vi "Open.vi"(7 "Allow multiple opens?":bool, 8 "error in (no error)":errorcluster, 10 "Channel Names":tag[](array[tag])) -> (0 "error out":errorcluster, 3 "Accelerometer Ref Out":T1)   [LabVIEW 2021, in "Accelerometer.lvlib"]
doc: "Opens a reference to one or more accelerometer channels. You must open a reference before you read values from an accelerometer channel."
uses:
  <vilib>/myRIO/Instrument Drivers/Onboard Devices/Accelerometer/Accelerometer.lvlib
  <vilib>/myRIO/Instrument Drivers/Onboard Devices/Accelerometer/typedefs/Accelerometer Reference.ctl
  <vilib>/myRIO/Common/Instrument Driver Framework/Utilities/typedefs/myRIO Generic Hardware Reference.ctl
  <vilib>/myRIO/Common/Instrument Driver Framework/Utilities/typedefs/Hardware Version Enum.ctl
  <vilib>/myRIO/Common/Instrument Driver Framework/Utilities/typedefs/myRIO v1.0 Reference.ctl
  <vilib>/myRIO/Common/Instrument Driver Framework/Utilities/typedefs/Generic FPGA Reference.ctl
  <vilib>/myRIO/Common/Instrument Driver Framework/myRIO v1.0/Accelerometer/typedefs/Accelerometer Channels List.ctl
  <vilib>/myRIO/Common/Instrument Driver Framework/myRIO v1.0/Accelerometer/typedefs/Accelerometer Channels Enum.ctl
  <vilib>/myRIO/Common/Instrument Driver Framework/Utilities/vis/Validate Channels.vi
  <vilib>/myRIO/Common/Instrument Driver Framework/myRIO v1.0/Accelerometer/vis/myRIO v1.0 Reserve Accelerometer.vi
  <vilib>/myRIO/Common/Instrument Driver Framework/roboRIO v1.0/Accelerometer/vis/roboRIO v1.0 Reserve Accelerometer.vi
  <vilib>/myRIO/Common/Instrument Driver Framework/myRIO v1.0/Resource Manager/vis/myRIO v1.0 Reserve Channel List.vi
  <vilib>/myRIO/Common/Instrument Driver Framework/myRIO v1.0/Accelerometer/vis/myRIO v1.0 Build MUX Configuration Accelerometer.vi
  <vilib>/myRIO/Common/Instrument Driver Framework/roboRIO v1.0/Resource Manager/vis/roboRIO v1.0 Reserve Channel List.vi
  <vilib>/myRIO/Common/Instrument Driver Framework/roboRIO v1.0/Accelerometer/vis/roboRIO v1.0 Build MUX Configuration Accelerometer.vi
  <vilib>/myRIO/Common/Instrument Driver Framework/myRIO v1.0/Resource Manager/vis/myRIO v1.0 Reserve Channel.vi
  <vilib>/myRIO/Common/Instrument Driver Framework/myRIO v1.0/Resource Manager/vis/myRIO v1.0 Unreserve Channel.vi
  <vilib>/myRIO/Common/Instrument Driver Framework/roboRIO v1.0/Resource Manager/vis/roboRIO v1.0 Reserve Channel.vi
  <vilib>/myRIO/Common/Instrument Driver Framework/roboRIO v1.0/Resource Manager/vis/roboRIO v1.0 Unreserve Channel.vi
  <vilib>/myRIO/Common/Instrument Driver Framework/myRIO v1.0/Resource Manager/vis/myRIO v1.0 Build Mutex Name.vi
  <vilib>/myRIO/Common/Instrument Driver Framework/roboRIO v1.0/Resource Manager/vis/roboRIO v1.0 Build Mutex Name.vi
  <vilib>/Utility/VariantDataType/GetNumericInfo.vi
  <vilib>/myRIO/Common/Instrument Driver Framework/myRIO v1.0/Accelerometer/vis/myRIO v1.0 Get Scaling Constant Accelerometer.vi
  <vilib>/myRIO/Common/Instrument Driver Framework/Utilities/vis/IO Manager.vi
  <vilib>/myRIO/Common/Instrument Driver Framework/Utilities/vis/Configuration Manager.vi
  <vilib>/myRIO/Common/Instrument Driver Framework/myRIO v1.0/myRIO v1.0 Close.vi
  <vilib>/myRIO/Common/Instrument Driver Framework/roboRIO v1.0/Accelerometer/vis/roboRIO v1.0 Get Scaling Constant Accelerometer.vi
  <vilib>/userdefined/High Color/nirio_resource_hc.ctl
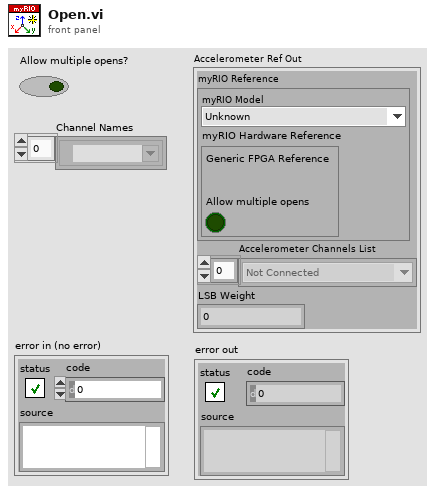
[diagram p1: front panel]
types:
  T1 = typedef "Accelerometer.lvlib/Accelerometer Reference.ctl" = cluster{"myRIO Reference":T2, "Accelerometer Channels List":T6, "LSB Weight":dbl}
  T2 = typedef "myRIO Generic Hardware Reference.ctl" = cluster{"myRIO Model":T3, "myRIO Hardware Reference":T4}
  T3 = typedef "Hardware Version Enum.ctl" = enum16{"Unknown", "myRIO-1900", "myRIO-1950", "roboRIO", "NI ELVIS RIO CM", "ELVIS III"}
  T4 = typedef "myRIO v1.0 Reference.ctl" = cluster{"Generic FPGA Reference":T5, "Allow multiple opens":bool}
  T5 = typedef "Generic FPGA Reference.ctl" = refnum<k20>
  T6 = typedef "Accelerometer Channels List.ctl" = T7[]
  T7 = typedef "Accelerometer Channels Enum.ctl" = enum16{"Not Connected", "X-Axis", "Y-Axis", "Z-Axis"}
  T8 = typedef "nirio_resource_hc.ctl" = tag
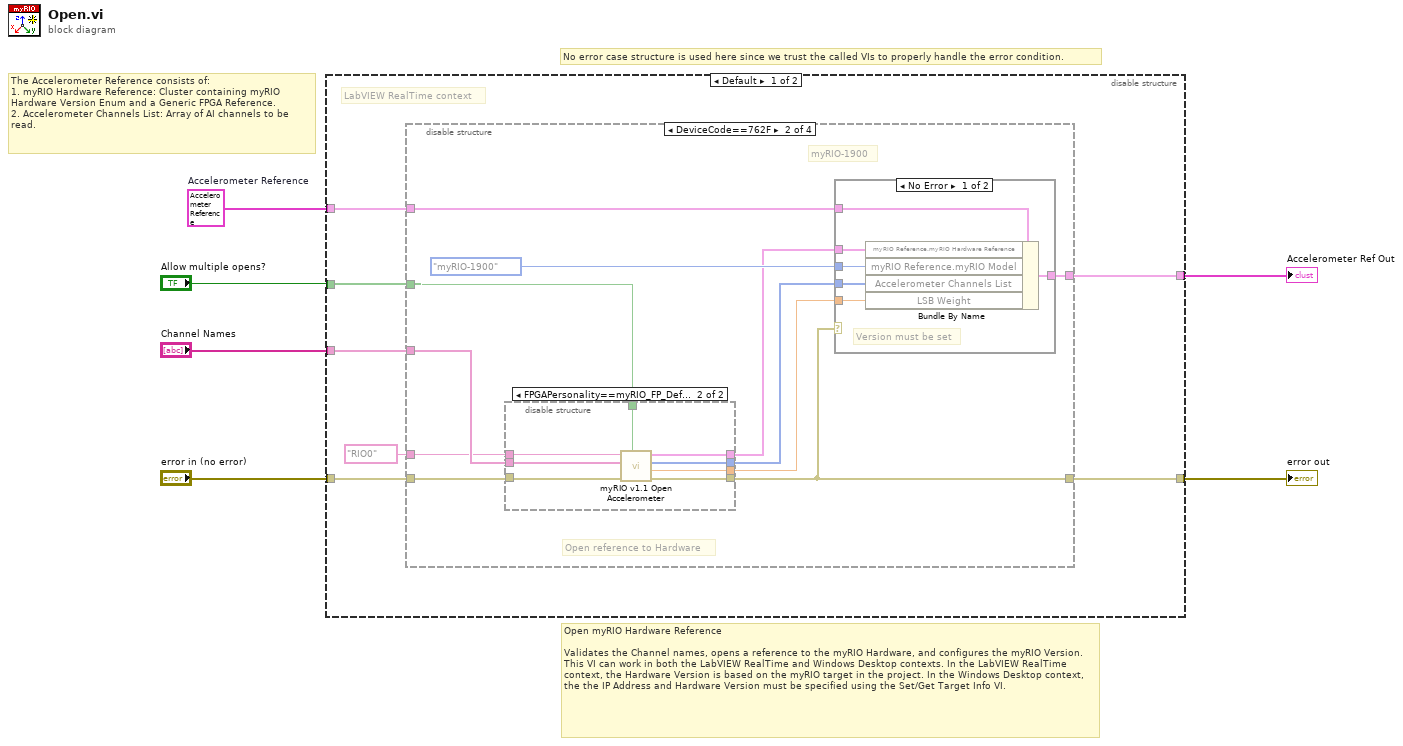
[diagram p0: block diagram]
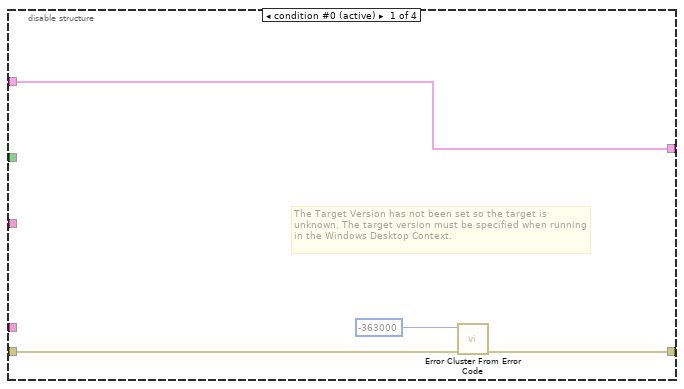
[diagram p2: hidden frame]
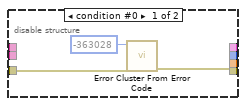
[diagram p3: hidden frame]
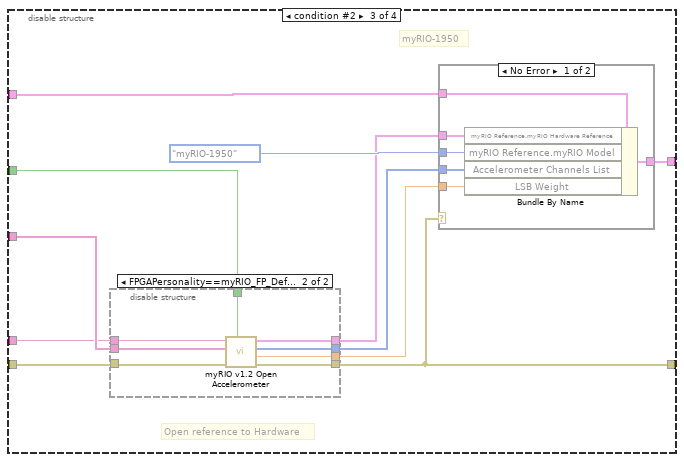
[diagram p5: hidden frame]
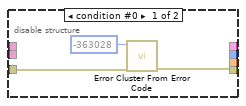
[diagram p6: hidden frame]
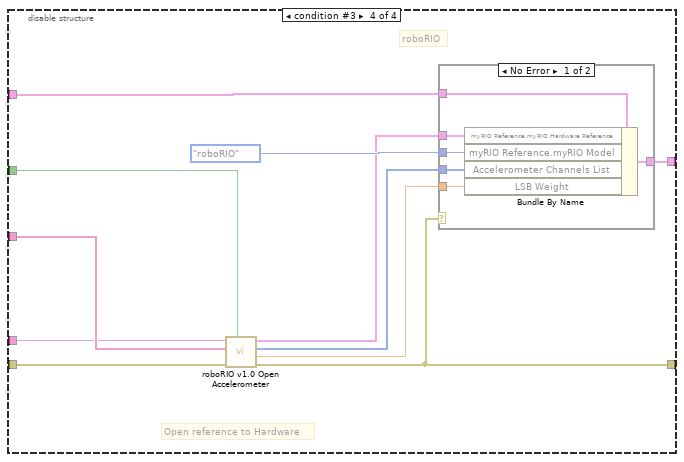
[diagram p8: hidden frame]
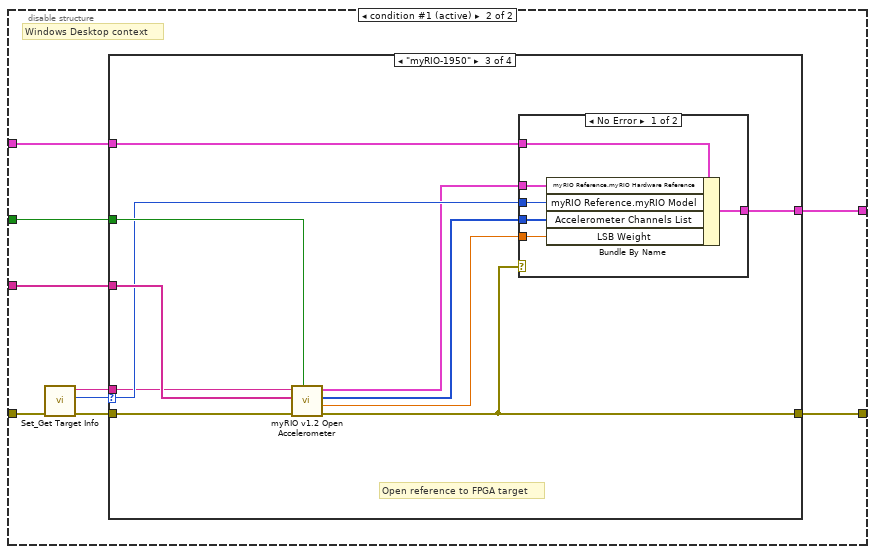
[diagram p10: hidden frame]
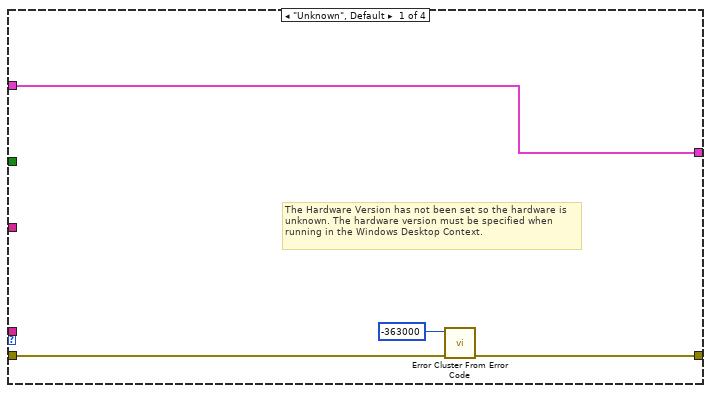
[diagram p11: hidden frame]
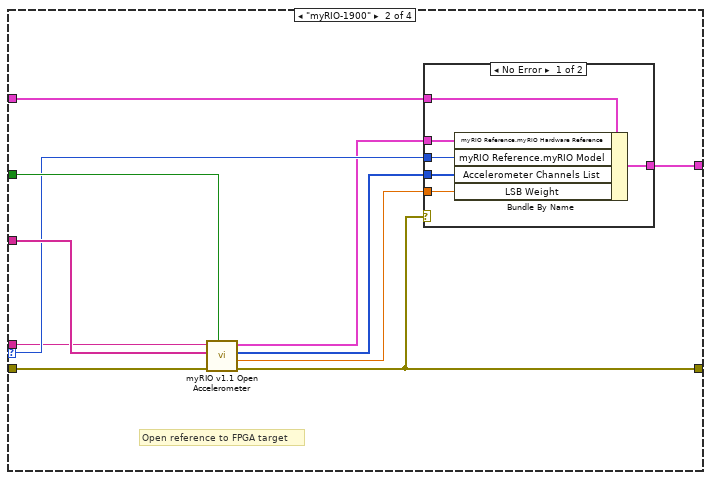
[diagram p12: hidden frame]
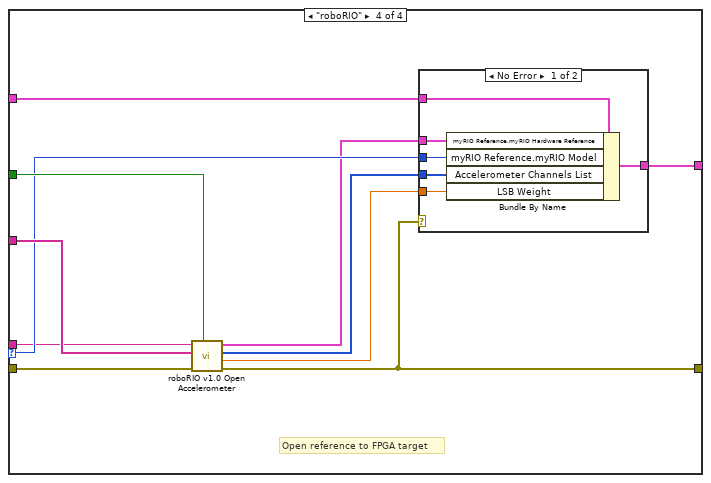
[diagram p15: hidden frame]
diagram:
  w3 = T1 {"myRIO Reference"={"myRIO Model"=enum."Unknown", "myRIO Hardware Reference"={"Generic FPGA Reference"=refnum, "Allow multiple opens"=FALSE}}, "Accelerometer Channels List"=[], "LSB Weight"=0.0}  # Accelerometer Reference
  # "No error case structure is used here since we trust the called VIs to properly handle the error condition."
  # "The Accelerometer Reference consists of:\n1. myRIO Hardware Reference: Cluster containing myRIO Hardware Version Enum and a Generic FPGA Reference.\n2. Accelerometer Channels List: Array of AI channels to be read."
  # "Open myRIO Hardware Reference\n\nValidates the Channel names, opens a reference to the myRIO Hardware, and configures the myRIO Version. This VI can work in both the LabVIEW RealTime and Windows Desktop contexts. In the LabVIEW RealTime context, the Hardware Version is based on the myRIO target in the project. In the Windows Desktop context, the the IP Address and Hardware Version must be specified using the Set/Get Target Info VI."
  n1 = disable-structure shown="Default" {
    disable-tunnel: [w13 w101] -> w4
    disable-tunnel: "Channel Names" -> [w12 w98]
    disable-tunnel: "Allow multiple opens?" -> [w11 w100]
    disable-tunnel: [w10 w99] -> w2
    disable-tunnel: "error in (no error)" -> [w9 w97]
    disable-tunnel: w3 -> [w8 w96]
    frame condition #0 {
      # "LabVIEW RealTime context"
      n2 = disable-structure shown="DeviceCode==762F" {
        disable-tunnel: [w17 w20 w48 w77] -> w13
        disable-tunnel: w12 -> [_ w28 w57 w86]
        disable-tunnel: w11 -> [_ w24 w56 w85]
        disable-tunnel: [w14 w27 w55 w84] -> w10
        disable-tunnel: w9 -> [w16 w25 w53 w82]
        disable-tunnel: w8 -> [w14 w23 w51 w80]
        disable-tunnel: T8 "RIO0" ("Resource name") -> [_ w21 w49 w78]
        frame condition #0 (active) {
          # "The Target Version has not been set so the target is unknown. The target version must be specified when running in the Windows Desktop Context."
          n3 = call <vilib>:"Error Cluster From Error Code.vi"("error in (no error)"=w16, "error code (0)"=-363000) -> ("error out"=w17:errorcluster)  [unwired: 7 in]
        }
        frame condition #1 {
          # "myRIO-1900"
          # "Open reference to Hardware"
          n4 = disable-structure shown="FPGAPersonality==myRIO_FP_Default, Default" {
            disable-tunnel: w28 -> [_ w39]
            disable-tunnel: w25 -> [w30 w38]
            disable-tunnel: w24 -> [_ w37]
            disable-tunnel: [_ w36] -> w22
            disable-tunnel: w21 -> [_ w35]
            disable-tunnel: [w29 w34] -> w20
            disable-tunnel: [_ w33] -> w19
            disable-tunnel: [_ w32] -> w18
            frame condition #0 {
              n5 = call <vilib>:"Error Cluster From Error Code.vi"("error in (no error)"=w30, "error code (0)"=-363028) -> ("error out"=w29:errorcluster)  [unwired: 7 in]
            }
            frame condition #1 (active) {
              n6 = call <vilib>:"myRIO v1.1 Open Accelerometer.vi"("Allow multiple opens?"=w37, "error in (no error)"=w38, "Channel Names"=w39, "Resource name"=w35) -> ("error out"=w34:errorcluster, "LSB Weight"=w32:dbl, "Accelerometer Channel List"=w36:T6, "myRIO Ref Out"=w33:T4)  [unwired: 4 in]
            }
          }
          n7 = case shown="No Error" w20 {
            tunnel: [w45 w46] -> w27
            tunnel: Hardware_Version_Enum."myRIO-1900" ("Hardware Version Enum") -> [w44 _]
            tunnel: w23 -> [w43 w46]
            tunnel: w22 -> [w42 _]
            tunnel: w19 -> [w41 _]
            tunnel: w18 -> [w40 _]
            frame No Error {
              # "Version must be set"
              n8 = Bundle By Name(cluster=w43, "myRIO Reference.myRIO Hardware Reference"=w41, "myRIO Reference.myRIO Model"=w44, "Accelerometer Channels List"=w42, "LSB Weight"=w40) -> (w45:T1)
            }
            frame Error {
            }
          }
        }
        frame condition #2 {
          # "myRIO-1950"
          # "Open reference to Hardware"
          n9 = disable-structure shown="FPGAPersonality==myRIO_FP_Default, Default" {
            disable-tunnel: w57 -> [_ w68]
            disable-tunnel: w56 -> [_ w67]
            disable-tunnel: w53 -> [w59 w66]
            disable-tunnel: [_ w65] -> w52
            disable-tunnel: [_ w64] -> w50
            disable-tunnel: w49 -> [_ w63]
            disable-tunnel: [w58 w62] -> w48
            disable-tunnel: [_ w61] -> w47
            frame condition #0 {
              n10 = call <vilib>:"Error Cluster From Error Code.vi"("error in (no error)"=w59, "error code (0)"=-363028) -> ("error out"=w58:errorcluster)  [unwired: 7 in]
            }
            frame condition #1 (active) {
              n11 = call <vilib>:"myRIO v1.2 Open Accelerometer.vi"("Allow multiple opens?"=w67, "error in (no error)"=w66, "Channel Names"=w68, "Resource name"=w63) -> ("error out"=w62:errorcluster, "LSB Weight"=w61:dbl, "Accelerometer Channel List"=w64:T6, "myRIO Ref Out"=w65:T4)  [unwired: 4 in]
            }
          }
          n12 = case shown="No Error" w48 {
            tunnel: [w74 w75] -> w55
            tunnel: Hardware_Version_Enum."myRIO-1950" ("Hardware Version Enum") -> [w73 _]
            tunnel: w52 -> [w70 _]
            tunnel: w51 -> [w72 w75]
            tunnel: w50 -> [w71 _]
            tunnel: w47 -> [w69 _]
            frame No Error {
              n13 = Bundle By Name(cluster=w72, "myRIO Reference.myRIO Hardware Reference"=w70, "myRIO Reference.myRIO Model"=w73, "Accelerometer Channels List"=w71, "LSB Weight"=w69) -> (w74:T1)
            }
            frame Error {
            }
          }
        }
        frame condition #3 {
          # "roboRIO"
          # "Open reference to Hardware"
          n14 = call <vilib>:"roboRIO v1.0 Open Accelerometer.vi"("Allow multiple opens?"=w85, "error in (no error)"=w82, "Channel Names"=w86, "Resource name"=w78) -> ("error out"=w77:errorcluster, "LSB Weight"=w76:dbl, "Accelerometer Channel List"=w79:T6, "myRIO Ref Out"=w81:T4)  [unwired: 4 in]
          n15 = case shown="No Error" w77 {
            tunnel: [w92 w93] -> w84
            tunnel: Hardware_Version_Enum."roboRIO" ("Hardware Version Enum") -> [w91 _]
            tunnel: w81 -> [w88 _]
            tunnel: w80 -> [w90 w93]
            tunnel: w79 -> [w89 _]
            tunnel: w76 -> [w87 _]
            frame No Error {
              n16 = Bundle By Name(cluster=w90, "myRIO Reference.myRIO Hardware Reference"=w88, "myRIO Reference.myRIO Model"=w91, "Accelerometer Channels List"=w89, "LSB Weight"=w87) -> (w92:T1)
            }
            frame Error {
            }
          }
        }
      }
    }
    frame condition #1 (active) {
      # "Windows Desktop context"
      n17 = call <vilib>:"Set_Get Target Info.vi"() -> ("Hardware Version"=w94:T3, "IP Address"=w95:string)  [unwired: 9 in, 1 out]
      n18 = case shown="\"myRIO-1950\"" w94 {
        selector: w94 -> [_ w113 w132 w150]
        tunnel: [w105 w108 w126 w144] -> w101
        tunnel: w98 -> [_ w116 w134 w152]
        tunnel: w100 -> [_ w115 w133 w151]
        tunnel: [w102 w114 w128 w146] -> w99
        tunnel: w97 -> [w103 w110 w131 w149]
        tunnel: w95 -> [_ w112 w130 w148]
        tunnel: w96 -> [w102 w111 w129 w147]
        frame "Unknown", Default {
          # "The Hardware Version has not been set so the hardware is unknown. The hardware version must be specified when running in the Windows Desktop Context."
          n19 = call <vilib>:"Error Cluster From Error Code.vi"("error in (no error)"=w103, "error code (0)"=-363000) -> ("error out"=w105:errorcluster)  [unwired: 7 in]
        }
        frame "myRIO-1900" {
          # "Open reference to FPGA target"
          n20 = call <vilib>:"myRIO v1.1 Open Accelerometer.vi"("Allow multiple opens?"=w115, "error in (no error)"=w110, "Channel Names"=w116, "Resource name"=w112) -> ("error out"=w108:errorcluster, "LSB Weight"=w106:dbl, "Accelerometer Channel List"=w109:T6, "myRIO Ref Out"=w107:T4)  [unwired: 4 in]
          n21 = case shown="No Error" w108 {
            tunnel: [w122 w123] -> w114
            tunnel: w113 -> [w121 _]
            tunnel: w111 -> [w120 w123]
            tunnel: w109 -> [w119 _]
            tunnel: w107 -> [w118 _]
            tunnel: w106 -> [w117 _]
            frame No Error {
              n22 = Bundle By Name(cluster=w120, "myRIO Reference.myRIO Hardware Reference"=w118, "myRIO Reference.myRIO Model"=w121, "Accelerometer Channels List"=w119, "LSB Weight"=w117) -> (w122:T1)
            }
            frame Error {
            }
          }
        }
        frame "myRIO-1950" {
          # "Open reference to FPGA target"
          n23 = call <vilib>:"myRIO v1.2 Open Accelerometer.vi"("Allow multiple opens?"=w133, "error in (no error)"=w131, "Channel Names"=w134, "Resource name"=w130) -> ("error out"=w126:errorcluster, "LSB Weight"=w124:dbl, "Accelerometer Channel List"=w127:T6, "myRIO Ref Out"=w125:T4)  [unwired: 4 in]
          n24 = case shown="No Error" w126 {
            tunnel: w132 -> [w140 _]
            tunnel: w129 -> [w139 w141]
            tunnel: [w138 w141] -> w128
            tunnel: w127 -> [w137 _]
            tunnel: w125 -> [w136 _]
            tunnel: w124 -> [w135 _]
            frame No Error {
              n25 = Bundle By Name(cluster=w139, "myRIO Reference.myRIO Hardware Reference"=w136, "myRIO Reference.myRIO Model"=w140, "Accelerometer Channels List"=w137, "LSB Weight"=w135) -> (w138:T1)
            }
            frame Error {
            }
          }
        }
        frame "roboRIO" {
          # "Open reference to FPGA target"
          n26 = call <vilib>:"roboRIO v1.0 Open Accelerometer.vi"("Allow multiple opens?"=w151, "error in (no error)"=w149, "Channel Names"=w152, "Resource name"=w148) -> ("error out"=w144:errorcluster, "LSB Weight"=w142:dbl, "Accelerometer Channel List"=w145:T6, "myRIO Ref Out"=w143:T4)  [unwired: 4 in]
          n27 = case shown="No Error" w144 {
            tunnel: w150 -> [w158 _]
            tunnel: w147 -> [w157 w159]
            tunnel: [w156 w159] -> w146
            tunnel: w145 -> [w155 _]
            tunnel: w143 -> [w154 _]
            tunnel: w142 -> [w153 _]
            frame No Error {
              n28 = Bundle By Name(cluster=w157, "myRIO Reference.myRIO Hardware Reference"=w154, "myRIO Reference.myRIO Model"=w158, "Accelerometer Channels List"=w155, "LSB Weight"=w153) -> (w156:T1)
            }
            frame Error {
            }
          }
        }
      }
    }
  }
  "Accelerometer Ref Out" <- w2
  "error out" <- w4
